vi "Wrap Angle.vi"(10 "Target Pitch (deg)":dbl) -> (2 "Correct Pitch":dbl)   [LabVIEW 2023]
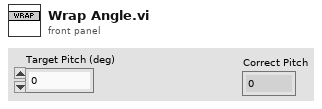
[diagram p1: front panel]
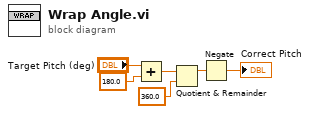
[diagram p0: block diagram]
diagram:
  n1 = Add(x="Target Pitch (deg)", y=180.0) -> (x+y=w4:dbl)
  n2 = Quotient & Remainder(x=w4, y=360.0) -> (x-y*floor(x/y)=w2:dbl)  [unwired: 1 out]
  n3 = Negate(x=w2) -> (-x=→"Correct Pitch":dbl)
